vi "Special_Function_Packet_Test.vi"() -> ()   [LabVIEW 2017]
uses:
  Controls/Control Packets/CM_Param.ctl
  Controls/Packet/Packet.ctl
  Controls/Packet/Packet_Direction.ctl
  Controls/Packet/Packet_Type.ctl
  Controls/Packet/Packet_Priority.ctl
  Controls/Control Packets/ES_Param.ctl
  Controls/Control Packets/RREQ_Param.ctl
  Controls/Connection Management/Connection_Management_Commands.ctl
panel:
  in  "Request FIDs":u8[](array[numeric])
  in  "Remote Request\nParameters":T1
  in  "Error and Status\nParameters":T2
  out "Execution status":string
  out "Network Error Status":T3(ring)
  in  "Number of tries":u32
  in  "Retry interval (ms)":u32
  in  "CM Packet In":T4
  in  "Connection Managemet\nParameters":T8
  in  "baud rate":u32=9600
  in  "COM Port In":refnum<visa-resource-name>
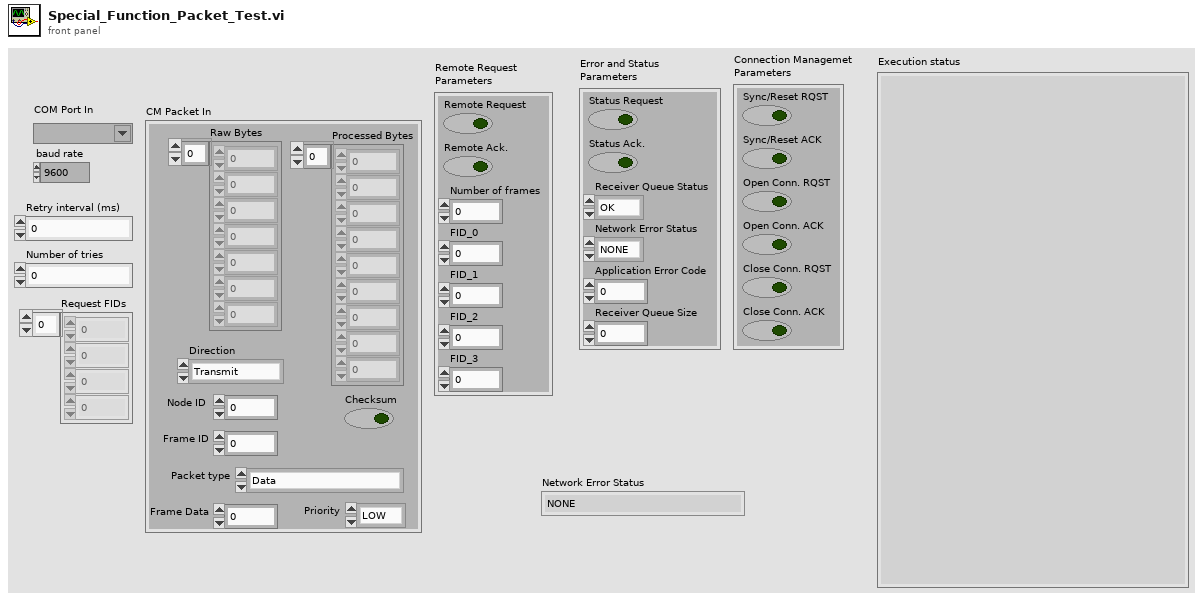
[diagram p1: front panel]
types:
  T1 = typedef "RREQ_Param.ctl" = cluster{"Remote Request":bool, "Remote Ack.":bool, "Number of frames":u8, "FID_0":u8, "FID_1":u8, "FID_2":u8, "FID_3":u8}
  T2 = typedef "ES_Param.ctl" = cluster{"Status Request":bool, "Status Ack.":bool, "Receiver Queue Status":enum16{"OK", "EMPTY", "FULL"}, "Network Error Status":enum16{"NONE", "CONNECTION_ALREADY_OPEN", "CONNECTION_ALREADY_CLOSED", "INVALID_FRAME_REQUEST"}, "Application Error Code":u16, "Receiver Queue Size":i32}
  T3 = enum16{"NONE", "CONNECTION_ALREADY_OPEN", "CONNECTION_ALREADY_CLOSED", "INVALID_FRAME_REQUEST"}
  T4 = typedef "Packet.ctl" = cluster{"Raw Bytes":u8[], "Checksum":bool, "Direction":T5, "Processed Bytes":u8[], "Node ID":u8, "Packet type":T6, "Frame Data":u32, "Priority":T7, "Frame ID":u8}
  T5 = typedef "Packet_Direction.ctl" = enum16{"Transmit", "Receive", "Bidirectional"}
  T6 = typedef "Packet_Type.ctl" = enum16{"Data", "Connection Management", "Remote Request", "Error/Status"}
  T7 = typedef "Packet_Priority.ctl" = enum16{"LOW", "HIGH"}
  T8 = typedef "CM_Param.ctl" = cluster{"Sync/Reset RQST":bool, "Sync/Reset ACK":bool, "Open Conn. RQST":bool, "Open Conn. ACK":bool, "Close Conn. RQST":bool, "Close Conn. ACK":bool}
  T9 = typedef "Connection_Management_Commands.ctl" = enum16{"Sync/Reset", "Open Connection", "Close Connection"}
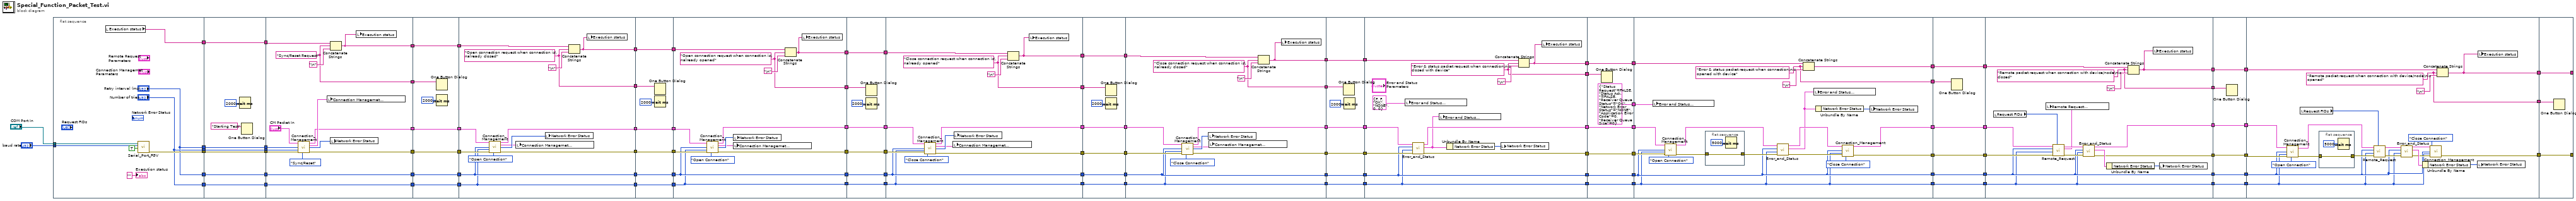
[diagram p0: block diagram]
diagram:
  n1 = flat-sequence {
    tunnel: "baud rate" -> [w114]
    tunnel: [w112] -> w105
    tunnel: ["Number of tries"] -> w103
    tunnel: ["Retry interval (ms)"] -> w101
    tunnel: [w110] -> w99
    tunnel: ["Retry interval (ms)"] -> w93
    tunnel: ["Number of tries"] -> w92
    tunnel: "COM Port In" -> [w107]
    tunnel: w105 -> [w122]
    tunnel: [w122] -> w104
    tunnel: w103 -> [w121]
    tunnel: [w121] -> w102
    tunnel: w101 -> [w118]
    tunnel: [w118] -> w100
    tunnel: w99 -> [w120]
    tunnel: [w120] -> w98
    tunnel: w93 -> [w117]
    tunnel: w92 -> [w116]
    tunnel: [w117] -> w91
    tunnel: [w116] -> w86
    tunnel: w104 -> [w137]
    tunnel: w102 -> [w134]
    tunnel: w100 -> [w133]
    tunnel: w98 -> [w128]
    tunnel: [w131] -> w97
    tunnel: [w130] -> w96
    tunnel: w91 -> [w126]
    tunnel: [w126] -> w89
    tunnel: [w125] -> w87
    tunnel: w86 -> [w125]
    tunnel: [w124] -> w85
    tunnel: [w123] -> w49
    tunnel: w97 -> [w144]
    tunnel: w96 -> [w143]
    tunnel: [w144] -> w95
    tunnel: [w143] -> w94
    tunnel: [w141] -> w90
    tunnel: w89 -> [w141]
    tunnel: [w140] -> w88
    tunnel: w87 -> [w140]
    tunnel: w85 -> [w139]
    tunnel: [w139] -> w84
    tunnel: w49 -> [w138]
    tunnel: w95 -> [w155]
    tunnel: w94 -> [w157]
    tunnel: w90 -> [w148]
    tunnel: w88 -> [w147]
    tunnel: w84 -> [w149]
    tunnel: [w153] -> w83
    tunnel: [w151] -> w82
    tunnel: [w146] -> w81
    tunnel: [w148] -> w77
    tunnel: [w147] -> w75
    tunnel: [w145] -> w48
    tunnel: w83 -> [w164]
    tunnel: w82 -> [w163]
    tunnel: w81 -> [w162]
    tunnel: [w164] -> w80
    tunnel: [w163] -> w79
    tunnel: [w162] -> w78
    tunnel: w77 -> [w160]
    tunnel: [w160] -> w76
    tunnel: w75 -> [w159]
    tunnel: [w159] -> w74
    tunnel: w48 -> [w158]
    tunnel: w80 -> [w176]
    tunnel: w79 -> [w177]
    tunnel: w78 -> [w169]
    tunnel: w76 -> [w167]
    tunnel: w74 -> [w166]
    tunnel: [w172] -> w73
    tunnel: [w171] -> w72
    tunnel: [w168] -> w71
    tunnel: [w167] -> w66
    tunnel: [w166] -> w64
    tunnel: [w165] -> w47
    tunnel: w73 -> [w184]
    tunnel: w72 -> [w183]
    tunnel: w71 -> [w182]
    tunnel: [w184] -> w69
    tunnel: [w183] -> w68
    tunnel: [w182] -> w67
    tunnel: w66 -> [w180]
    tunnel: [w180] -> w65
    tunnel: w64 -> [w179]
    tunnel: [w179] -> w63
    tunnel: w47 -> [w178]
    tunnel: w69 -> [w196]
    tunnel: w68 -> [w197]
    tunnel: w67 -> [w189]
    tunnel: w65 -> [w187]
    tunnel: w63 -> [w186]
    tunnel: [w192] -> w62
    tunnel: [w191] -> w61
    tunnel: [w188] -> w60
    tunnel: [w187] -> w56
    tunnel: [w186] -> w54
    tunnel: [w185] -> w46
    tunnel: w62 -> [w204]
    tunnel: w61 -> [w203]
    tunnel: w60 -> [w202]
    tunnel: [w204] -> w59
    tunnel: [w203] -> w58
    tunnel: [w202] -> w57
    tunnel: w56 -> [w200]
    tunnel: [w200] -> w55
    tunnel: w54 -> [w199]
    tunnel: [w199] -> w53
    tunnel: w46 -> [w198]
    tunnel: w59 -> [w216]
    tunnel: w58 -> [w217]
    tunnel: w57 -> [w209]
    tunnel: w55 -> [w206]
    tunnel: w53 -> [w205]
    tunnel: [w212] -> w52
    tunnel: [w211] -> w51
    tunnel: [w208] -> w50
    tunnel: [w207] -> w45
    tunnel: [w206] -> w40
    tunnel: [w205] -> w39
    tunnel: w52 -> [w224]
    tunnel: w51 -> [w223]
    tunnel: w50 -> [w222]
    tunnel: w45 -> [w220]
    tunnel: [w224] -> w44
    tunnel: [w223] -> w43
    tunnel: [w222] -> w42
    tunnel: [w219] -> w41
    tunnel: w40 -> [w219]
    tunnel: w39 -> [w218]
    tunnel: [w218] -> w38
    tunnel: w44 -> [w236]
    tunnel: w43 -> [w237]
    tunnel: w42 -> [w229]
    tunnel: w41 -> [w226]
    tunnel: w38 -> [w225]
    tunnel: [w234] -> w37
    tunnel: [w231] -> w36
    tunnel: [w228] -> w35
    tunnel: [w227] -> w34
    tunnel: [w226] -> w30
    tunnel: [w225] -> w28
    tunnel: w37 -> [w244]
    tunnel: w36 -> [w243]
    tunnel: w35 -> [w242]
    tunnel: w34 -> [w241]
    tunnel: [w244] -> w33
    tunnel: [w243] -> w32
    tunnel: [w242] -> w31
    tunnel: w30 -> [w240]
    tunnel: [w240] -> w29
    tunnel: w28 -> [w239]
    tunnel: [w239] -> w27
    tunnel: [T2 {"Status Request"=FALSE, "Status Ack."=FALSE, "Receiver Queue Status"=enum."OK", "Network Error Status"=enum."NONE", "Application Error Code"=0, "Receiver Queue Size"=0} ("Cluster")] -> w11
    tunnel: w33 -> [w263]
    tunnel: w32 -> [w264]
    tunnel: w31 -> [w250]
    tunnel: w29 -> [w247]
    tunnel: w27 -> [w246]
    tunnel: [w256] -> w26
    tunnel: [w254] -> w25
    tunnel: [w249] -> w24
    tunnel: [w248] -> w23
    tunnel: [w247] -> w19
    tunnel: [w246] -> w17
    tunnel: w11 -> [w245]
    tunnel: w26 -> [w272]
    tunnel: w25 -> [w271]
    tunnel: w24 -> [w270]
    tunnel: w23 -> [w269]
    tunnel: [w272] -> w22
    tunnel: [w271] -> w21
    tunnel: [w270] -> w20
    tunnel: w19 -> [w268]
    tunnel: [w268] -> w18
    tunnel: w17 -> [w267]
    tunnel: [w267] -> w16
    tunnel: w22 -> [w287]
    tunnel: w21 -> [w288]
    tunnel: w20 -> [w277]
    tunnel: w18 -> [w274]
    tunnel: w16 -> [w273]
    tunnel: [w280] -> w15
    tunnel: [w279] -> w14
    tunnel: [w276] -> w13
    tunnel: [w275] -> w12
    tunnel: [w274] -> w7
    tunnel: [w273] -> w5
    tunnel: w15 -> [w294]
    tunnel: w14 -> [w293]
    tunnel: w13 -> [w292]
    tunnel: w12 -> [w291]
    tunnel: [w294] -> w10
    tunnel: [w293] -> w9
    tunnel: [w291] -> w8
    tunnel: w7 -> [w290]
    tunnel: [w290] -> w6
    tunnel: w5 -> [w289]
    tunnel: [w289] -> w4
    tunnel: w10 -> [w314]
    tunnel: w9 -> [w315]
    tunnel: w8 -> [w297]
    tunnel: w6 -> [w301]
    tunnel: w4 -> [w300]
    tunnel: [w299] -> w3
    tunnel: [w295] -> w2
    tunnel: [w296] -> w1
    tunnel: [w320] -> _
    tunnel: w3 -> [w320]
    tunnel: w2 -> [w318]
    tunnel: w1 -> [w319]
    tunnel: [w318] -> _
    frame #0 {
      n2 = local read "Execution status"() -> (w110:string)
      n3 = call "Serial_Port_FGV.vi"("Initialize ?"=TRUE, "baud rate"=w114, "COM Port In"=w107) -> ("error out"=w112:errorcluster)  [unwired: 7 in, 1 out]
      "Execution status" <- "" ("Execution status")
    }
    frame #1 {
      n4 = Wait (ms)(milliseconds to wait=u32 2000) -> ()  [unwired: 1 out]
      n5 = One Button Dialog(message="Starting Test") -> ()  [unwired: 1 in, 1 out]
    }
    frame #2 {
      w123 = "Sync/Reset Request" ("string")
      n6 = call "Connection_Management.vi"("CM Packet In"="CM Packet In", "Commands"=Connection_Management_Commands."Sync/Reset", "Retry interval (ms)"=w133, "Number of tries"=w134, "error in (no error)"=w137) -> ("CM Packet Out"=w131:T4, "CM Params Out"=w132:T8, "Network Error Status"=w129:T3, "error out"=w130:errorcluster)  [unwired: 7 in]
      n7 = local write "Connection Managemet\nParameters"(w132) -> ()
      n8 = Concatenate Strings(w128, w123, "\n") -> (w124:string)
      n9 = local write "Network Error Status"(w129) -> ()
      n10 = local write "Execution status"(w124) -> ()
    }
    frame #3 {
      n11 = One Button Dialog(message=w138) -> ()  [unwired: 1 in, 1 out]
      n12 = Wait (ms)(milliseconds to wait=u32 2000) -> ()  [unwired: 1 out]
    }
    frame #4 {
      w145 = "Open connection request when connection is\nalready closed" ("string")
      n13 = call "Connection_Management.vi"("CM Packet In"=w155, "Commands"=Connection_Management_Commands."Open Connection", "Retry interval (ms)"=w148, "Number of tries"=w147, "error in (no error)"=w157) -> ("CM Packet Out"=w153:T4, "CM Params Out"=w152:T8, "Network Error Status"=w154:T3, "error out"=w151:errorcluster)  [unwired: 7 in]
      n14 = local write "Connection Managemet\nParameters"(w152) -> ()
      n15 = local write "Network Error Status"(w154) -> ()
      n16 = Concatenate Strings(w149, w145, "\n") -> (w146:string)
      n17 = local write "Execution status"(w146) -> ()
    }
    frame #5 {
      n18 = One Button Dialog(message=w158) -> ()  [unwired: 1 in, 1 out]
      n19 = Wait (ms)(milliseconds to wait=u32 2000) -> ()  [unwired: 1 out]
    }
    frame #6 {
      w165 = "Open connection request when connection is\nalready opened" ("string")
      n20 = call "Connection_Management.vi"("CM Packet In"=w176, "Commands"=Connection_Management_Commands."Open Connection", "Retry interval (ms)"=w167, "Number of tries"=w166, "error in (no error)"=w177) -> ("CM Packet Out"=w172:T4, "CM Params Out"=w173:T8, "Network Error Status"=w174:T3, "error out"=w171:errorcluster)  [unwired: 7 in]
      n21 = local write "Connection Managemet\nParameters"(w173) -> ()
      n22 = local write "Network Error Status"(w174) -> ()
      n23 = Concatenate Strings(w169, w165, "\n") -> (w168:string)
      n24 = local write "Execution status"(w168) -> ()
    }
    frame #7 {
      n25 = One Button Dialog(message=w178) -> ()  [unwired: 1 in, 1 out]
      n26 = Wait (ms)(milliseconds to wait=u32 2000) -> ()  [unwired: 1 out]
    }
    frame #8 {
      w185 = "Close connection request when connection is\nalready opened" ("string")
      n27 = call "Connection_Management.vi"("CM Packet In"=w196, "Commands"=Connection_Management_Commands."Close Connection", "Retry interval (ms)"=w187, "Number of tries"=w186, "error in (no error)"=w197) -> ("CM Packet Out"=w192:T4, "CM Params Out"=w193:T8, "Network Error Status"=w194:T3, "error out"=w191:errorcluster)  [unwired: 7 in]
      n28 = local write "Connection Managemet\nParameters"(w193) -> ()
      n29 = local write "Network Error Status"(w194) -> ()
      n30 = Concatenate Strings(w189, w185, "\n") -> (w188:string)
      n31 = local write "Execution status"(w188) -> ()
    }
    frame #9 {
      n32 = One Button Dialog(message=w198) -> ()  [unwired: 1 in, 1 out]
      n33 = Wait (ms)(milliseconds to wait=u32 2000) -> ()  [unwired: 1 out]
    }
    frame #10 {
      w207 = "Close connection request when connection is\nalready closed" ("string")
      n34 = call "Connection_Management.vi"("CM Packet In"=w216, "Commands"=Connection_Management_Commands."Close Connection", "Retry interval (ms)"=w206, "Number of tries"=w205, "error in (no error)"=w217) -> ("CM Packet Out"=w212:T4, "CM Params Out"=w213:T8, "Network Error Status"=w214:T3, "error out"=w211:errorcluster)  [unwired: 7 in]
      n35 = local write "Network Error Status"(w214) -> ()
      n36 = local write "Connection Managemet\nParameters"(w213) -> ()
      n37 = Concatenate Strings(w209, w207, "\n") -> (w208:string)
      n38 = local write "Execution status"(w208) -> ()
    }
    frame #11 {
      n39 = One Button Dialog(message=w220) -> ()  [unwired: 1 in, 1 out]
      n40 = Wait (ms)(milliseconds to wait=u32 2000) -> ()  [unwired: 1 out]
    }
    frame #12 {
      w227 = "Error & status packet request when connection\nis closed with device" ("string")
      n41 = local write "Error and Status\nParameters"(T2 {"Status Request"=FALSE, "Status Ack."=FALSE, "Receiver Queue Status"=enum."OK", "Network Error Status"=enum."NONE", "Application Error Code"=0, "Receiver Queue Size"=0} ("Error and Status\nParameters")) -> ()
      n42 = call "Error_and_Status.vi"("error in (no error)"=w237, "Retry interval (ms)"=w225, "Number of tries"=w226, "ES Packet"=w236) -> ("error out"=w231:errorcluster, "ES Param Out"=w232:T2, "ES Packet Out"=w234:T4)  [unwired: 5 in]
      n43 = local write "Error and Status\nParameters"(w232) -> ()
      n44 = Unbundle By Name(w232) -> ("Network Error Status"=w235:T3)
      n45 = local write "Network Error Status"(w235) -> ()
      n46 = Concatenate Strings(w229, w227, "\n") -> (w228:string)
      n47 = local write "Execution status"(w228) -> ()
    }
    frame #13 {
      n48 = One Button Dialog(message=w241) -> ()  [unwired: 1 in, 1 out]
    }
    frame #14 {
      w248 = "Error & status packet request when connection\nis opened with device" ("string")
      n49 = local write "Error and Status\nParameters"(w245) -> ()
      n50 = call "Connection_Management.vi"("CM Packet In"=w263, "Commands"=Connection_Management_Commands."Open Connection", "Retry interval (ms)"=w247, "Number of tries"=w246, "error in (no error)"=w264) -> ("CM Packet Out"=w259:T4, "error out"=w261:errorcluster)  [unwired: 7 in, 2 out]
      n51 = flat-sequence {
        tunnel: w261 -> [w266]
        tunnel: [w266] -> w260
        frame #0 {
          n52 = Wait (ms)(milliseconds to wait=u32 5000) -> ()  [unwired: 1 out]
        }
      }
      n53 = call "Error_and_Status.vi"("error in (no error)"=w260, "Retry interval (ms)"=w246, "Number of tries"=w247, "ES Packet"=w259) -> ("error out"=w258:errorcluster, "ES Param Out"=w253:T2, "ES Packet Out"=w257:T4)  [unwired: 5 in]
      n54 = Concatenate Strings(w250, w248, "\n") -> (w249:string)
      n55 = local write "Error and Status\nParameters"(w253) -> ()
      n56 = Unbundle By Name(w253) -> ("Network Error Status"=w252:T3)
      n57 = call "Connection_Management.vi"("CM Packet In"=w257, "Commands"=Connection_Management_Commands."Close Connection", "Retry interval (ms)"=w247, "Number of tries"=w246, "error in (no error)"=w258) -> ("CM Packet Out"=w256:T4, "error out"=w254:errorcluster)  [unwired: 7 in, 2 out]
      n58 = local write "Network Error Status"(w252) -> ()
    }
    frame #15 {
      n59 = One Button Dialog(message=w269) -> ()  [unwired: 1 in, 1 out]
    }
    frame #16 {
      w276 = "Remote packet request when connection with device/node\nis closed" ("string")
      n60 = local read "Request FIDs"() -> (w286:u8[])
      n61 = call "Remote_Request.vi"("FIDs"=w286, "error in (no error)"=w288, "Retry interval (ms)"=w273, "Number of tries"=w274, "RREQ Packet"=w287) -> ("error out"=w284:errorcluster, "RREQ Param Out"=w281:T1, "RREQ Packet Out"=w285:T4)  [unwired: 3 in, 1 out]
      n62 = local write "Remote Request\nParameters"(w281) -> ()
      n63 = call "Error_and_Status.vi"("error in (no error)"=w284, "Retry interval (ms)"=w273, "Number of tries"=w274, "ES Packet"=w285) -> ("error out"=w279:errorcluster, "ES Param Out"=w283:T2, "ES Packet Out"=w280:T4)  [unwired: 5 in]
      n64 = Unbundle By Name(w283) -> ("Network Error Status"=w282:T3)
      n65 = Concatenate Strings(w277, w276, "\n") -> (w275:string)
      n66 = local write "Execution status"(w275) -> ()
      n67 = local write "Network Error Status"(w282) -> ()
    }
    frame #17 {
      n68 = One Button Dialog(message=w292) -> ()  [unwired: 1 in, 1 out]
    }
    frame #18 {
      w296 = "Remote packet request when connection with device/node\nis opened" ("string")
      n69 = call "Connection_Management.vi"("CM Packet In"=w314, "Commands"=Connection_Management_Commands."Open Connection", "Retry interval (ms)"=w301, "Number of tries"=w300, "error in (no error)"=w315) -> ("CM Packet Out"=w310:T4, "error out"=w312:errorcluster)  [unwired: 7 in, 2 out]
      n70 = local read "Request FIDs"() -> (w309:u8[])
      n71 = flat-sequence {
        tunnel: w312 -> [w316]
        tunnel: [w316] -> w311
        frame #0 {
          n72 = Wait (ms)(milliseconds to wait=u32 5000) -> ()  [unwired: 1 out]
        }
      }
      n73 = call "Remote_Request.vi"("FIDs"=w309, "error in (no error)"=w311, "Retry interval (ms)"=w300, "Number of tries"=w301, "RREQ Packet"=w310) -> ("error out"=w308:errorcluster, "RREQ Packet Out"=w307:T4)  [unwired: 3 in, 2 out]
      n74 = call "Error_and_Status.vi"("error in (no error)"=w308, "Retry interval (ms)"=w300, "Number of tries"=w301, "ES Packet"=w307) -> ("error out"=w304:errorcluster, "ES Param Out"=w306:T2, "ES Packet Out"=w303:T4)  [unwired: 5 in]
      n75 = Unbundle By Name(w306) -> ("Network Error Status"=w305:T3)
      n76 = call "Connection_Management.vi"("CM Packet In"=w303, "Commands"=Connection_Management_Commands."Close Connection", "Retry interval (ms)"=w301, "Number of tries"=w300, "error in (no error)"=w304) -> ("error out"=w299:errorcluster)  [unwired: 7 in, 3 out]
      n77 = Concatenate Strings(w297, w296, "\n") -> (w295:string)
      n78 = local write "Network Error Status"(w305) -> ()
      n79 = local write "Execution status"(w295) -> ()
    }
    frame #19 {
      n80 = One Button Dialog(message=w319) -> ()  [unwired: 1 in, 1 out]
    }
  }
